vi "Read Voltage.vi"(4 "entrée d'erreur (pas d'erreur)":errorcluster) -> (0 "sortie d'erreur":errorcluster, 3 "tension":dbl format="%.2f")   [LabVIEW 2009]
doc: "Ce VI est utilisé dans les cours LabVIEW Fondamental 1 et 2.\n\nCe VI simule un relevé de mesures de tension avec une carte DAQ. Utilisez ce VI au lieu du VI Express Assistant DAQ dans tous les exercices de ce cours qui mesurent des températures. Ce VI est un sous-VI de tous les exercices de démonstration."
panel:
  in  "mesures":dbl[](array[numeric])=[163.0, 163.0, 163.0, 163.0, 163.0, 163.0, 165.0, 169.0, 172.0, 173.0, 172.0, 172.0, 171.0, 171.0, 174.0, 176.0, 177.0, 178.0, 178.0, 179.0, 178.0, 177.0, 176.0, 175.0, 175.0, 174.0, 173.0, 172.0, 172.0, 172.0, 172.0, 172.0, 171.0, 171.0, 170.0, 170.0, 170.0, 172.0, 173.0, 174.0, 175.0, 177.0, 178.0, 178.0, 178.0, 177.0, 176.0, 175.0, 176.0, 178.0, 179.0, 180.0, 179.0, 178.0, 178.0, 176.0, 176.0, 176.0, 174.0, 174.0, 174.0, 173.0, 173.0, 175.0, 176.0, 178.0, 178.0, 177.0, 176.0, 175.0, 175.0, 174.0, 174.0, 173.0, 173.0, 172.0, 172.0, 171.0, 171.0, 170.0, 170.0, 170.0, 170.0, 170.0, 170.0, 170.0, 169.0, 166.0, 167.0, 169.0, 170.0, 169.0, 168.0, 168.0, 168.0, 168.0, 167.0, 167.0, 167.0, 167.0] format="%.2f"
  # "*Ce VI représente un VI qui lit la tension \nsur la voie 0 du périphérique 1 et applique \nun facteur de 100 sur le signal pour le \nconvertir en température.*"
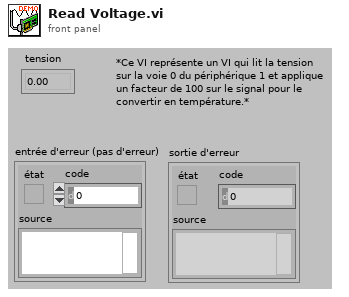
[diagram p1: front panel]
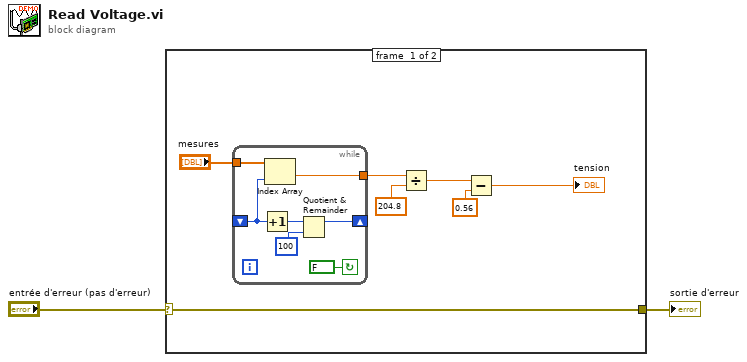
[diagram p0: block diagram]
diagram:
  n1 = case "Structure Condition" shown="Pas d'erreur" "entrée d'erreur (pas d'erreur)" {
    selector: "entrée d'erreur (pas d'erreur)" -> [w4 w17]
    tunnel: [w4 w17] -> w1
    frame #0 {
      n2 = while "Boucle While" {
        tunnel: "mesures" -> [w11]
        tunnel: [w12] -> w7
        shift-left: _ -> [w16]
        shift-right: [w13] -> _
        stop <- FALSE continue-if-true
        n3 = Increment(x=w16) -> (x+1=w15:i32)
        n4 = Index Array(array=w11, index=w16) -> (element=w12:dbl)
        n5 = Quotient & Remainder(x=w15, y=100) -> (x-y*floor(x/y)=w13:i32)  [unwired: 1 out]
      }
      n6 = Divide ("Diviser")(x=w7, y=204.8) -> (x/y=w6:dbl)
      n7 = Subtract ("Soustraire")(x=w6, y=0.56) -> (x-y=→"tension":dbl)
    }
    frame #1 {
    }
  }
  "sortie d'erreur" <- w1
